vi "Dialog GraphSetting (XY).vi"(11 "XYグラフref(in)":refnum<vi>) -> ()   [LabVIEW 2016]
uses:
  TypeDef/GraphSetting Appearance.ctl
  TypeDef/GraphSetting Plot.ctl
  SupportVIs/GraphSetting Scale.ctl
  TypeDef/GraphSetting DisplayFormatType.ctl
  TypeDef/GraphSetting All.ctl
  TypeDef/GraphSetting Command.ctl
  Library/Event/Write User Event (Array).vi
  <vilib>/Utility/xml.llb/Write to XML File(string).vi
  <vilib>/Utility/xml.llb/Read From XML File(string).vi
  <vilib>/measure/NI_MABase.lvlib
  TypeDef/XYData.ctl
panel:
  out "XYグラフ":cluster{"X":dbl[], "Y":dbl[]}[](graph)
  in  "ファイル読込":bool
  in  "ファイル保存":bool
  in  "タブ制御器":enum32{"外観", "スケール", "プロット"}(tab)
  in  "外観":T1
  in  "Yスケール選択":u16(ring) items=["振幅"]
  in  "スケール(Y軸)":T2
  in  "スケール(X軸)":T2
  in  "Xスケール選択":u16(ring) items=["時間"]
  in  "プロット":T4 {"Yスケール" items=["振幅"]; "Xスケール" items=["時間"]; "プロット補間" max=5 step=1; "ポイントスタイル" max=16 step=1; "太さ" max=5 step=1; "ラインスタイル" max=4 step=1}
  in  "プロット選択":u16(ring) items=["正弦波", "プロット1"]
  in  "停止ボタン":bool
  # "スケールのスタイルとカラー"
  # "スケール係数"
  # "スケールのスタイルとカラー"
  # "スケールのスタイルとカラー"
  # "スケール係数"
  # "スケールのスタイルとカラー"
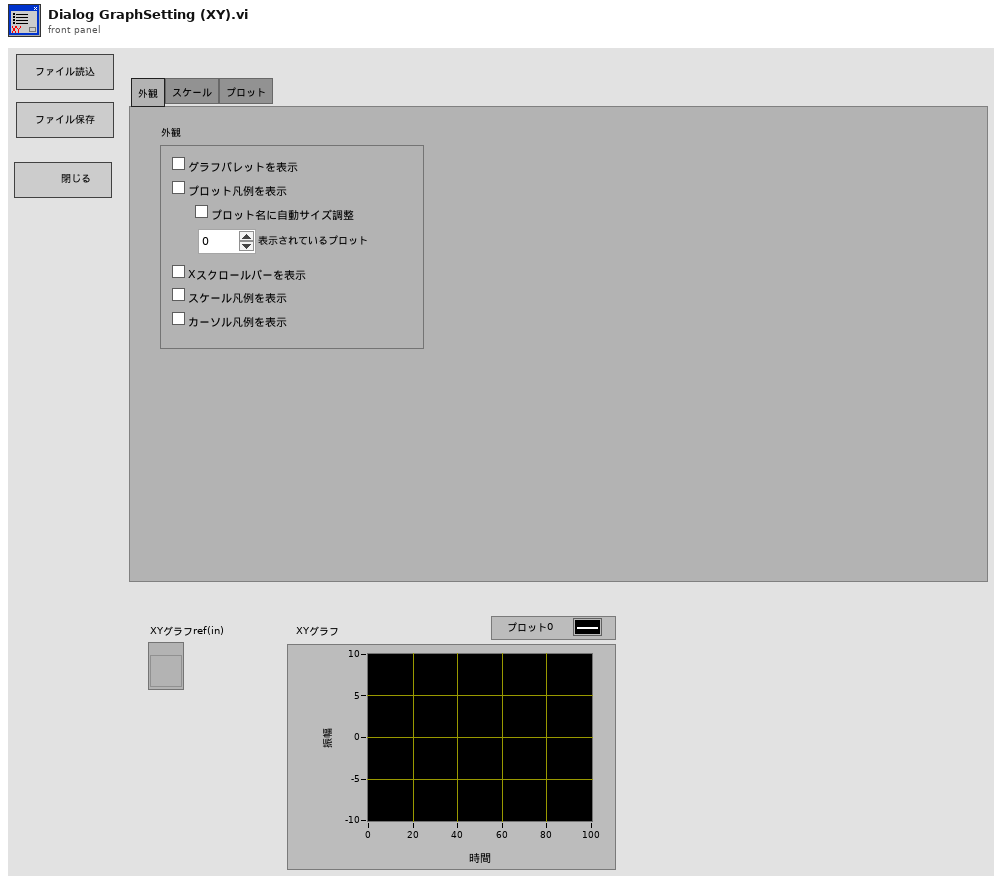
[diagram p1: front panel]
types:
  T1 = typedef "GraphSetting Appearance.ctl" = cluster{"グラフパレットを表示":bool, "プロット凡例を表示":bool, "プロット名に自動サイズ調整":bool, "表示されているプロット":u32, "Xスクロールバーを表示":bool, "スケール凡例を表示":bool, "カーソル凡例を表示":bool}
  T2 = typedef "GraphSetting Scale.ctl" = cluster{"名前":string, "スケールラベルを表示":bool, "スケールを表示":bool, "ログ":bool, "反転":bool, "自動スケール":bool, "最小":dbl, "最大":dbl, "オフセット":dbl, "乗数":dbl, "主目盛り":u32, "補助目盛り":u32, "マーカテキスト":u32, "主グリッド":u32, "補助グリッド":u32, "タイプ":T3, "小数点以下桁数":u8}
  T3 = typedef "GraphSetting DisplayFormatType.ctl" = enum8{"浮動小数点", "科学", "工学", "バイナリ", "８進数", "１６進数", "相対時間", "時間と日時", "SI"}
  T4 = typedef "GraphSetting Plot.ctl" = cluster{"名前":string, "表示":bool, "ラインスタイル":u8, "太さ":u8, "ポイントスタイル":u8, "プロット補間":u8, "ラインカラー":u32, "ポイント/塗りつぶし":u32, "Xスケール":u16, "Yスケール":u16}
  T5 = typedef "XYData.ctl" = cluster{"X":dbl[], "Y":dbl[]}
  T6 = typedef "GraphSetting All.ctl" = cluster{"外観":T1, "スケールX[]":T2[], "スケールY[]":T2[], "プロット[]":T4[]}
  T7 = typedef "GraphSetting Command.ctl" = enum16{"Get(ref->ctl)", "Set(ctl->ref)"}
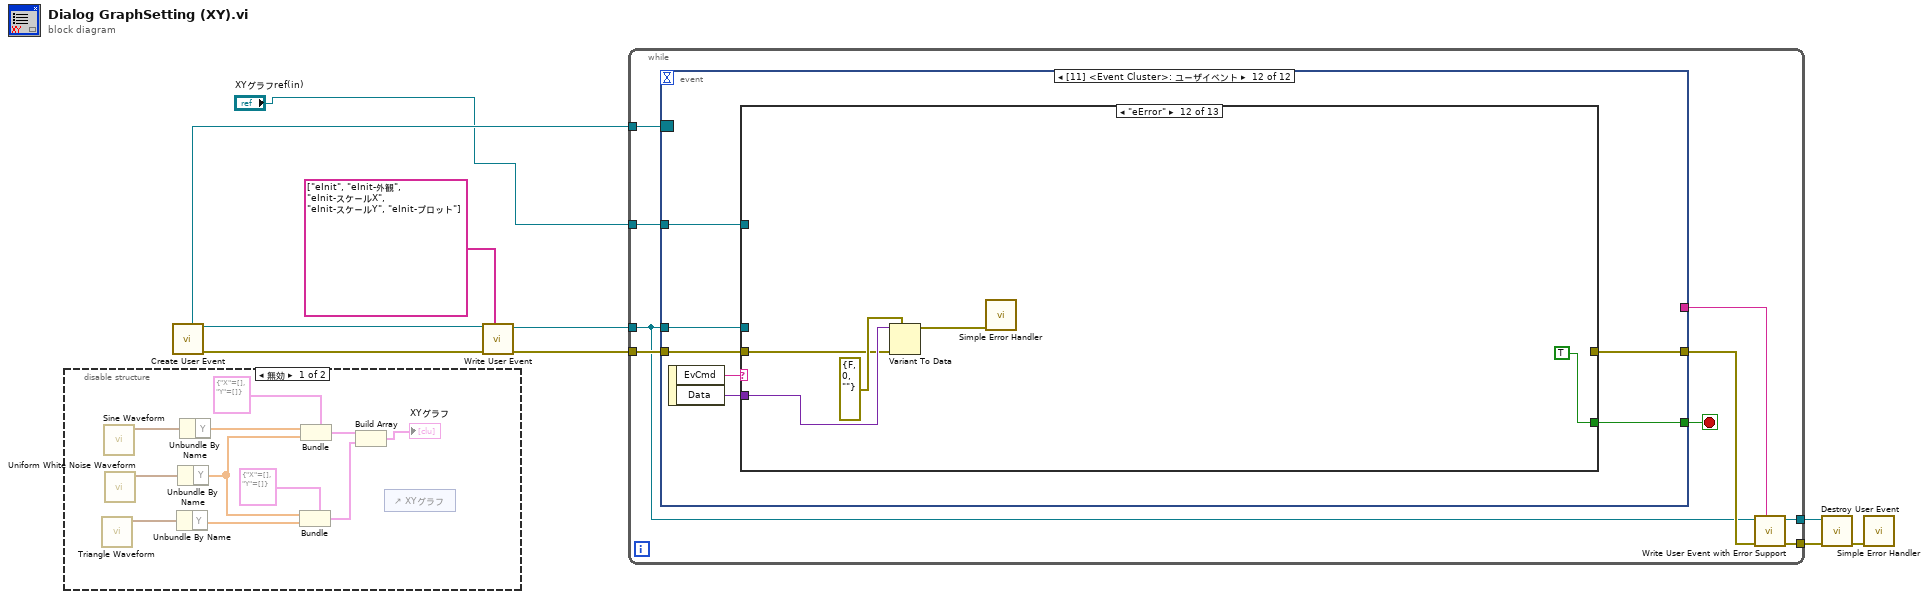
[diagram p0: block diagram]
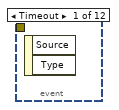
[diagram p3: hidden frame]
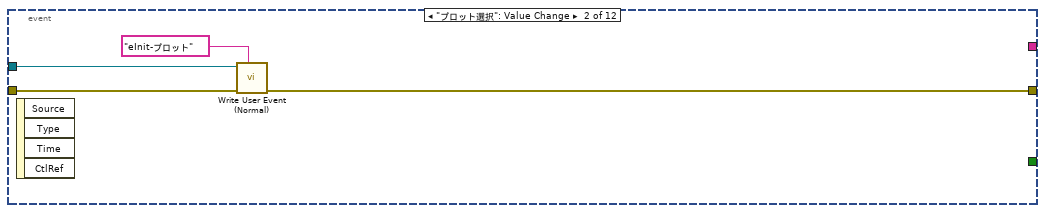
[diagram p4: hidden frame]
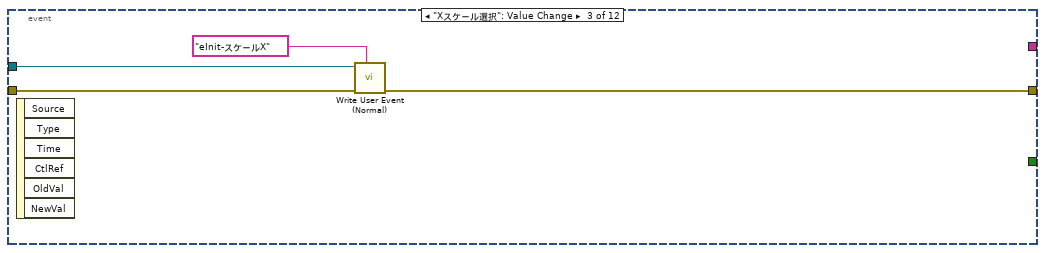
[diagram p5: hidden frame]
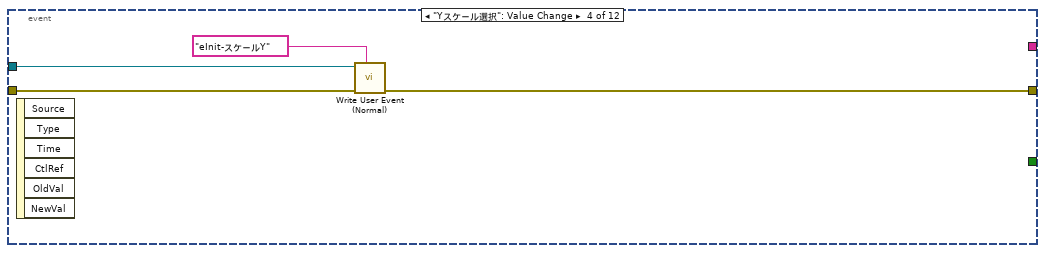
[diagram p6: hidden frame]
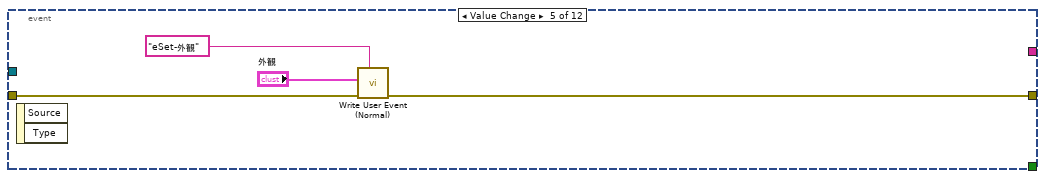
[diagram p7: hidden frame]
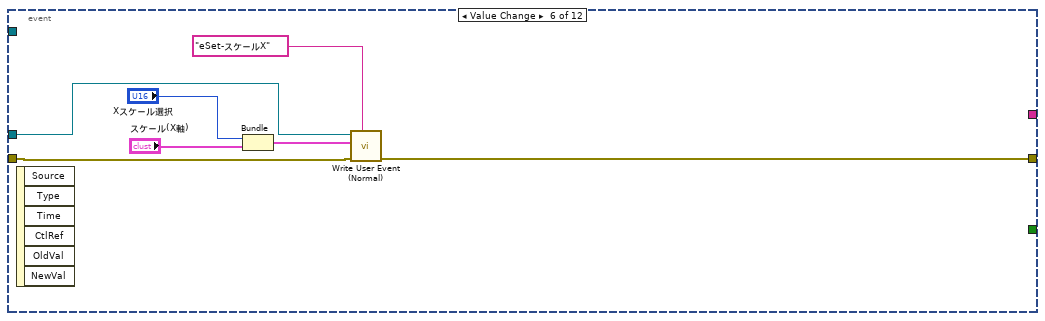
[diagram p8: hidden frame]
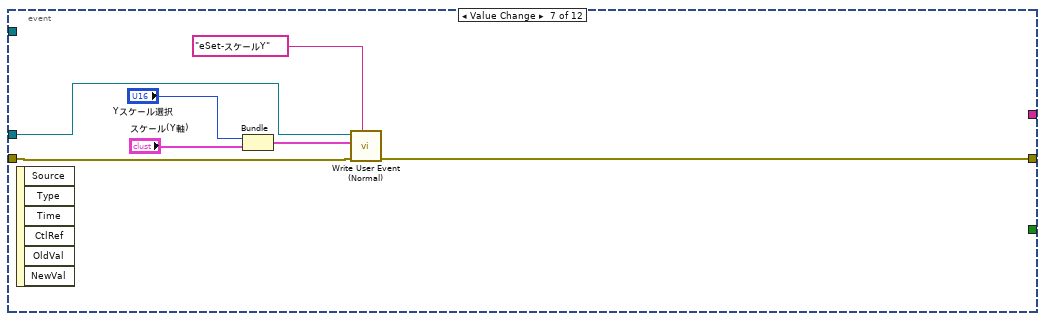
[diagram p9: hidden frame]
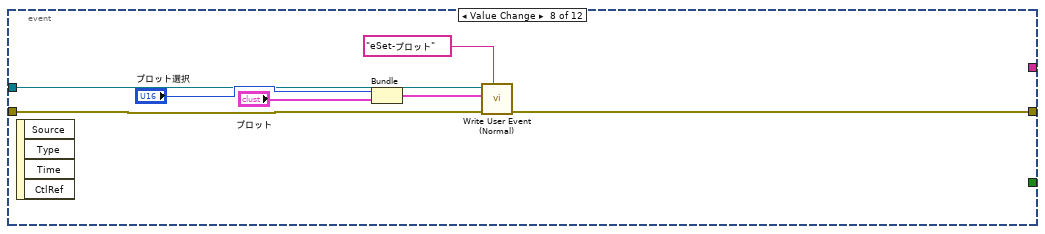
[diagram p10: hidden frame]
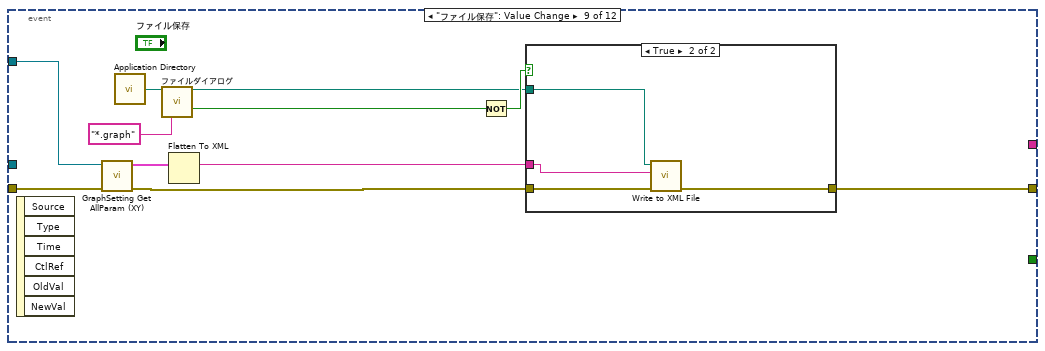
[diagram p11: hidden frame]
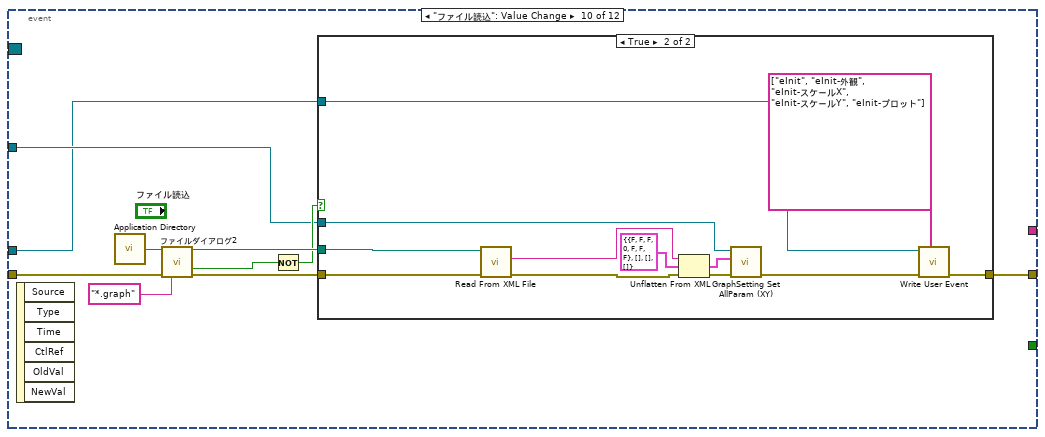
[diagram p13: hidden frame]
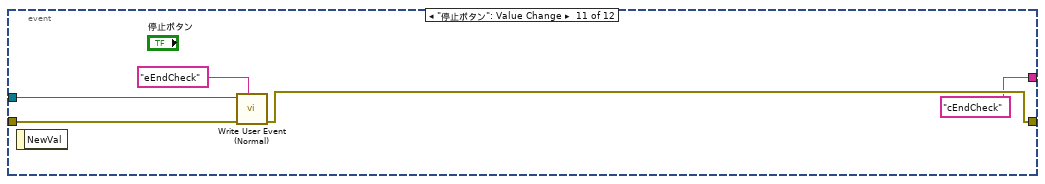
[diagram p15: hidden frame]
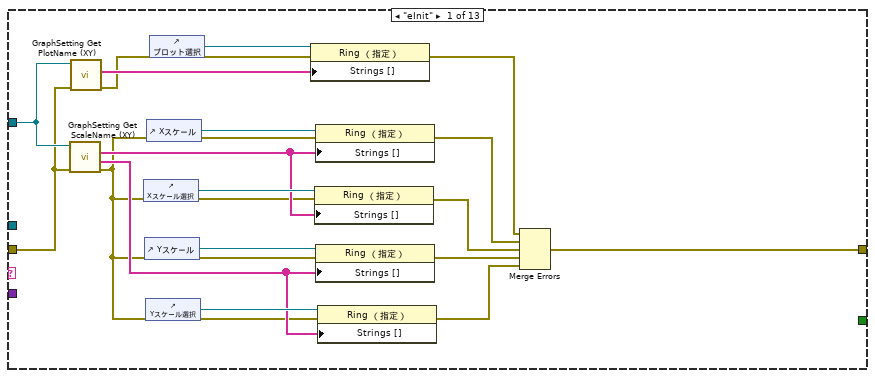
[diagram p16: hidden frame]
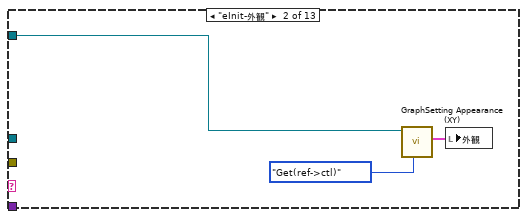
[diagram p17: hidden frame]
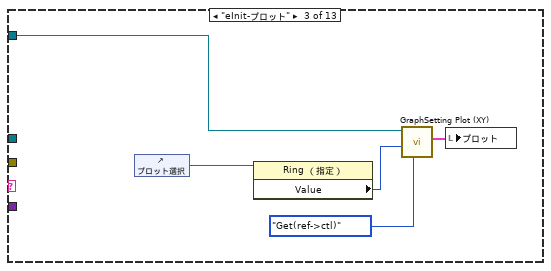
[diagram p18: hidden frame]
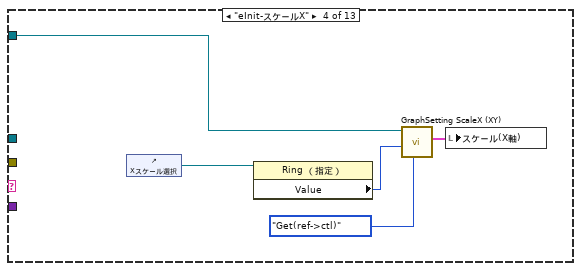
[diagram p19: hidden frame]
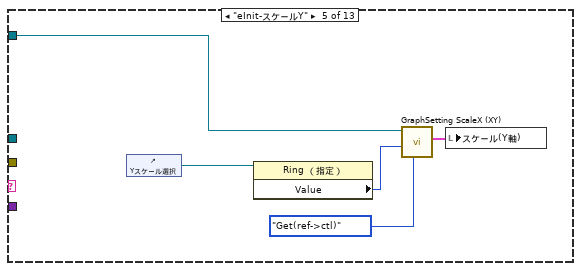
[diagram p20: hidden frame]
diagram:
  n1 = disable-structure shown="無効" {
    frame Disabled {
      n2 = call <vilib>:"Triangle Waveform.vi"() -> ("signal out"=w16:waveform(dbl))  [unwired: 10 in, 1 out]
      n3 = call <vilib>:"Sine Waveform.vi"() -> ("signal out"=w21:waveform(dbl))  [unwired: 10 in, 1 out]
      n4 = call <vilib>:"Uniform White Noise Waveform.vi"() -> ("signal out"=w17:waveform(dbl))  [unwired: 10 in, 1 out]
      n5 = Unbundle By Name(w16) -> ("Y"=w14:dbl[])
      n6 = Unbundle By Name(w17) -> ("Y"=w13:dbl[])
      n7 = Unbundle By Name(w21) -> ("Y"=w18:dbl[])
      n8 = Bundle(cluster=T5 {"X"=[], "Y"=[]} ("XYグラグデータ"), "X"=w13, "Y"=w14) -> (w11:T5)
      n9 = Bundle(cluster=T5 {"X"=[], "Y"=[]} ("XYグラグデータ"), "X"=w18, "Y"=w13) -> (w12:T5)
      n10 = Build Array(w12, w11) -> (→"XYグラフ":T5[])
      n11 = control-ref of="XYグラフ"() -> ()  [unwired: 1 out]
    }
    frame Enabled {
    }
  }
  n12 = call "Create User Event.vi"() -> ("error out"=w8:errorcluster, "User Event"=w9:refnum<user-event>, "Event Registration Refnum"=w10:refnum<event-registration>)  [unwired: 9 in]
  n13 = call-poly "Write User Event.vi"("EvCmd[]"=string[] ["eInit", "eInit-外観", "eInit-スケールX", "eInit-スケールY", "eInit-プロット"], "エラー入力（エラーなし）"=w8, "ユーザイベント入力"=w9) -> ("エラー出力"=w4:errorcluster, "ユーザイベント出力"=w5:refnum<user-event>)  [unwired: 7 in]
  n14 = while {
    tunnel: w4 -> [w29]
    tunnel: w10 -> [w30]
    tunnel: [w26] -> w7
    tunnel: w5 -> [w22]
    tunnel: "XYグラフref(in)" -> [w28]
    tunnel: [w23] -> w2
    stop <- w24 stop-if-true
    n15 = event shown="[11] <Event Cluster>: ユーザイベント" {
      selector: w30 -> [_ _ _ _ _ _ _ _ _ _ _ _]
      dyn-events: _ -> [_ _ _ _ _ _ _ _ _ _ _ _]
      timeout: _ -> [_ _ _ _ _ _ _ _ _ _ _ _]
      tunnel: [_ _ _ _ _ _ _ _ _ _ _ w114] -> w24
      tunnel: [_ w32 w36 w39 w43 w48 w55 w62 w72 w85 w108 w115] -> w27
      tunnel: w29 -> [_ w33 w38 w41 w44 w47 w56 w63 w69 w91 w110 w116]
      tunnel: w22 -> [_ w34 w37 w40 _ w51 w57 w64 _ w84 w111 w113]
      tunnel: w28 -> [_ _ _ _ _ _ _ _ w68 w86 _ w112]
      tunnel: [_ _ _ _ _ _ _ _ _ _ "cEndCheck" _] -> w25
      event Timeout {
        n16 = event-data() -> ()  [unwired: 1 in, 2 out]
      }
      event "プロット選択": Value Change {
        n17 = event-data() -> ()  [unwired: 1 in, 4 out]
        n18 = call "Write User Event (Normal).vi"("EvCmd"="eInit-プロット", "エラー入力（エラーなし）"=w33, "ユーザイベント入力"=w34) -> ("エラー出力"=w32:errorcluster)  [unwired: 7 in, 1 out]
      }
      event "Xスケール選択": Value Change {
        n19 = event-data() -> ()  [unwired: 1 in, 6 out]
        n20 = call "Write User Event (Normal).vi"("EvCmd"="eInit-スケールX", "エラー入力（エラーなし）"=w38, "ユーザイベント入力"=w37) -> ("エラー出力"=w36:errorcluster)  [unwired: 7 in, 1 out]
      }
      event "Yスケール選択": Value Change {
        n21 = event-data() -> ()  [unwired: 1 in, 6 out]
        n22 = call "Write User Event (Normal).vi"("EvCmd"="eInit-スケールY", "エラー入力（エラーなし）"=w41, "ユーザイベント入力"=w40) -> ("エラー出力"=w39:errorcluster)  [unwired: 7 in, 1 out]
      }
      event Value Change {
        n23 = event-data() -> ()  [unwired: 1 in, 2 out]
        n24 = call "Write User Event (Normal).vi"("EvCmd"="eSet-外観", "エラー入力（エラーなし）"=w44, "データ"="外観") -> ("エラー出力"=w43:errorcluster)  [unwired: 7 in, 1 out]
      }
      event Value Change {
        n25 = event-data() -> ()  [unwired: 1 in, 6 out]
        n26 = Bundle("Xスケール選択"="Xスケール選択", "スケール(X軸)"="スケール(X軸)") -> (w52:cluster{"Xスケール選択":u16, "スケール(X軸)":T2})  [unwired: 1 in]
        n27 = call "Write User Event (Normal).vi"("EvCmd"="eSet-スケールX", "エラー入力（エラーなし）"=w47, "データ"=w52, "ユーザイベント入力"=w51) -> ("エラー出力"=w48:errorcluster)  [unwired: 6 in, 1 out]
      }
      event Value Change {
        n28 = event-data() -> ()  [unwired: 1 in, 6 out]
        n29 = Bundle("Yスケール選択"="Yスケール選択", "スケール(Y軸)"="スケール(Y軸)") -> (w58:cluster{"Yスケール選択":u16, "スケール(Y軸)":T2})  [unwired: 1 in]
        n30 = call "Write User Event (Normal).vi"("EvCmd"="eSet-スケールY", "エラー入力（エラーなし）"=w56, "データ"=w58, "ユーザイベント入力"=w57) -> ("エラー出力"=w55:errorcluster)  [unwired: 6 in, 1 out]
      }
      event Value Change {
        n31 = event-data() -> ()  [unwired: 1 in, 4 out]
        n32 = Bundle("プロット選択"="プロット選択", "プロット"="プロット") -> (w65:cluster{"プロット選択":u16, "プロット":T4})  [unwired: 1 in]
        n33 = call "Write User Event (Normal).vi"("EvCmd"="eSet-プロット", "エラー入力（エラーなし）"=w63, "データ"=w65, "ユーザイベント入力"=w64) -> ("エラー出力"=w62:errorcluster)  [unwired: 6 in, 1 out]
      }
      event "ファイル保存": Value Change {
        n34 = event-data() -> ()  [unwired: 1 in, 6 out]
        n35 = call "GraphSetting Get AllParam (XY).vi"("エラー入力（エラーなし）"=w69, "XYグラフref(in)"=w68) -> ("エラー出力"=w71:errorcluster, "クラスタ"=w70:cluster{"外観(out)":T1, T2[], T2[], T4[]})  [unwired: 8 in]
        n36 = call <vilib>:"Application Directory.vi"() -> ("Application Directory"=w77:path)
        n37 = call "ファイルダイアログ"("start path"=w77, "pattern (all files)"="*.graph") -> ("selected path"=w73:path, "cancelled"=w74:bool)  [unwired: 10 in, 2 out]
        n38 = Flatten To XML(anything=w70) -> (xml string=w75:string)
        n39 = Not(x=w74) -> (.not. x?=w76:bool)
        n40 = case shown="TRUE" w76 {
          tunnel: w73 -> [_ w83]
          tunnel: w75 -> [_ w82]
          tunnel: w71 -> [w79 w80]
          tunnel: [w79 w81] -> w72
          frame False {
          }
          frame True {
            n41 = call-poly <vilib>:"Write to XML File.vi"("error in (no error)"=w80, "XML Input"=w82, "XML File Path"=w83) -> ("error out"=w81:errorcluster)  [unwired: 6 in, 2 out]
          }
        }
      }
      event "ファイル読込": Value Change {
        n42 = event-data() -> ()  [unwired: 1 in, 6 out]
        n43 = call <vilib>:"Application Directory.vi"() -> ("Application Directory"=w93:path)
        n44 = call "ファイルダイアログ2"("start path"=w93, "error in"=w91, "pattern (all files)"="*.graph") -> ("selected path"=w90:path, "cancelled"=w89:bool, "error out"=w87:errorcluster)  [unwired: 9 in, 1 out]
        n45 = Not(x=w89) -> (.not. x?=w88:bool)
        n46 = case shown="TRUE" w88 {
          tunnel: w90 -> [_ w104]
          tunnel: w87 -> [w94 w102]
          tunnel: w86 -> [_ w99]
          tunnel: [w94 w96] -> w85
          tunnel: w84 -> [_ w98]
          frame False {
          }
          frame True {
            n47 = call-poly <vilib>:"Read From XML File.vi"("error in (no error)"=w102, "XML File Path"=w104) -> ("error out"=w103:errorcluster, "XML Elements"=w105:string)  [unwired: 7 in, 1 out]
            n48 = Unflatten From XML(xml string=w105, type=T6 {"外観"={"グラフパレットを表示"=FALSE, "プロット凡例を表示"=FALSE, "プロット名に自動サイズ調整"=FALSE, "表示されているプロット"=0, "Xスクロールバーを表示"=FALSE, "スケール凡例を表示"=FALSE, "カーソル凡例を表示"=FALSE}, "スケールX[]"=[], "スケールY[]"=[], "プロット[]"=[]} ("出力クラスタ"), error in (no error)=w103) -> (value=w101:T6, error out=w100:errorcluster)
            n49 = call "GraphSetting Set AllParam (XY).vi"("error in (no error)"=w100, "Chartグラフパラメータ"=w101, "XYグラフref(in)"=w99) -> ("error out"=w97:errorcluster)  [unwired: 8 in]
            n50 = call-poly "Write User Event.vi"("EvCmd[]"=string[] ["eInit", "eInit-外観", "eInit-スケールX", "eInit-スケールY", "eInit-プロット"], "エラー入力（エラーなし）"=w97, "ユーザイベント入力"=w98) -> ("エラー出力"=w96:errorcluster)  [unwired: 7 in, 1 out]
          }
        }
      }
      event "停止ボタン": Value Change {
        n51 = event-data() -> ()  [unwired: 1 in, 1 out]
        n52 = call "Write User Event (Normal).vi"("EvCmd"="eEndCheck", "エラー入力（エラーなし）"=w110, "ユーザイベント入力"=w111) -> ("エラー出力"=w108:errorcluster)  [unwired: 7 in, 1 out]
      }
      event User Event {
        n53 = event-data() -> ("EvCmd"=w118:string, "Data"=w117:variant)  [unwired: 1 in]
        n54 = case shown="\"eError\"" w118 {
          selector: w118 -> [_ _ _ _ _ _ _ _ _ _ _ _ w202]
          tunnel: w117 -> [_ _ _ _ _ w159 w167 w178 w188 _ _ w201 _]
          tunnel: w116 -> [w128 _ _ _ _ w157 w169 w177 w187 w192 w196 w199 _]
          tunnel: [w119 _ _ _ _ w155 w162 w171 w181 w191 w196 _ _] -> w115
          tunnel: [_ _ _ _ _ _ _ _ _ _ TRUE TRUE _] -> w114
          tunnel: w113 -> [_ _ _ _ _ _ _ _ _ w194 _ _ _]
          tunnel: w112 -> [w131 w139 w144 w149 w154 w160 w163 w175 w185 _ _ _ _]
          frame "eInit" {
            n55 = call "GraphSetting Get ScaleName (XY).vi"("error in (no error)"=w128, "XYグラフref(in)"=w131) -> ("error out"=w125:errorcluster, "Y軸名称[]"=w127:string[], "X軸名称[]"=w134:string[])  [unwired: 7 in]
            n56 = call "GraphSetting Get PlotName (XY).vi"("error in (no error)"=w128, "XYグラフref(in)"=w131) -> ("error out"=w126:errorcluster, "プロット名称[]"=w129:string[])  [unwired: 8 in]
            n57 = control-ref of="Xスケール選択"() -> (w135:refnum<vi>)
            n58 = control-ref of="Yスケール"() -> (w132:refnum<vi>)
            n59 = control-ref of="Yスケール選択"() -> (w133:refnum<vi>)
            n60 = control-ref of="Xスケール"() -> (w136:refnum<vi>)
            n61 = control-ref of="プロット選択"() -> (w130:refnum<vi>)
            n62 = property class="Ring （指定）"(reference=w130, error in=w126, "Strings []"=w129) -> (error out=w124:errorcluster)  [unwired: 1 out]
            n63 = property class="Ring （指定）"(reference=w135, error in=w125, "Strings []"=w134) -> (error out=w122:errorcluster)  [unwired: 1 out]
            n64 = property class="Ring （指定）"(reference=w136, error in=w125, "Strings []"=w134) -> (error out=w123:errorcluster)  [unwired: 1 out]
            n65 = property class="Ring （指定）"(reference=w132, error in=w125, "Strings []"=w127) -> (error out=w121:errorcluster)  [unwired: 1 out]
            n66 = property class="Ring （指定）"(reference=w133, error in=w125, "Strings []"=w127) -> (error out=w120:errorcluster)  [unwired: 1 out]
            n67 = Merge Errors(w124, w123, w122, w121, w120) -> (w119:errorcluster)
          }
          frame "eInit-外観" {
            n68 = call "GraphSetting Appearance (XY).vi"("コマンド"=GraphSetting_Command."Get(ref->ctl)", "XYグラフref(in)"=w139) -> ("外観(out)"=w138:T1)  [unwired: 8 in, 1 out]
            n69 = local write "外観"(w138) -> ()
          }
          frame "eInit-プロット" {
            n70 = control-ref of="プロット選択"() -> (w143:refnum<vi>)
            n71 = property class="Ring （指定）"(reference=w143) -> ("Value"=w142:u16)  [unwired: 1 in, 2 out]
            n72 = call "GraphSetting Plot (XY).vi"("コマンド"=GraphSetting_Command."Get(ref->ctl)", "アクティブプロット"=w142, "XYグラフref(in)"=w144) -> ("プロット(out)"=w140:T4)  [unwired: 7 in, 1 out]
            n73 = local write "プロット"(w140) -> ()
          }
          frame "eInit-スケールX" {
            n74 = control-ref of="Xスケール選択"() -> (w148:refnum<vi>)
            n75 = property class="Ring （指定）"(reference=w148) -> ("Value"=w147:u16)  [unwired: 1 in, 2 out]
            n76 = call "GraphSetting ScaleX (XY).vi"("コマンド"=GraphSetting_Command."Get(ref->ctl)", "アクティブスケール(X)"=w147, "XYグラフref(in)"=w149) -> ("スケール(out)"=w145:T2)  [unwired: 7 in, 1 out]
            n77 = local write "スケール(X軸)"(w145) -> ()
          }
          frame "eInit-スケールY" {
            n78 = control-ref of="Yスケール選択"() -> (w153:refnum<vi>)
            n79 = property class="Ring （指定）"(reference=w153) -> ("Value"=w152:u16)  [unwired: 1 in, 2 out]
            n80 = call "GraphSetting ScaleX (XY).vi"("コマンド"=GraphSetting_Command."Get(ref->ctl)", "アクティブスケール(X)"=w152, "XYグラフref(in)"=w154) -> ("スケール(out)"=w150:T2)  [unwired: 7 in, 1 out]
            n81 = local write "スケール(Y軸)"(w150) -> ()
          }
          frame "eSet-外観" {
            n82 = Variant To Data(error in=w157, Variant=w159) -> (data=w158:T1, error out=w156:errorcluster)  [unwired: 1 in]
            n83 = call "GraphSetting Appearance (XY).vi"("コマンド"=GraphSetting_Command."Set(ctl->ref)", "error in (no error)"=w156, "外観(in)"=w158, "XYグラフref(in)"=w160) -> ("error out"=w155:errorcluster)  [unwired: 6 in, 1 out]
          }
          frame "eSet-スケールX" {
            n84 = Variant To Data(type=cluster{"Xスケール選択":u16, "スケール(X軸)":T2} {"Xスケール選択"=0, "スケール(X軸)"={"名前"="", "スケールラベルを表示"=FALSE, "スケールを表示"=FALSE, "ログ"=FALSE, "反転"=FALSE, "自動スケール"=FALSE, "最小"=0.0, "最大"=0.0, "オフセット"=0.0, "乗数"=0.0, "主目盛り"=0, "補助目盛り"=0, "マーカテキスト"=0, "主グリッド"=0, "補助グリッド"=0, "タイプ"=enum."浮動小数点", "小数点以下桁数"=0}} ("出力クラスタ"), Variant=w167) -> (data=w166:cluster{"Xスケール選択":u16, "スケール(X軸)":T2})  [unwired: 1 in, 1 out]
            n85 = Unbundle(w166) -> ("Xスケール選択"=w164:u16, "スケール(X軸)"=w165:T2)
            n86 = call "GraphSetting ScaleX (XY).vi"("コマンド"=GraphSetting_Command."Set(ctl->ref)", "error in (no error)"=w169, "アクティブスケール(X)"=w164, "スケール(in)"=w165, "XYグラフref(in)"=w163) -> ("error out"=w162:errorcluster)  [unwired: 5 in, 1 out]
          }
          frame "eSet-スケールY" {
            n87 = Variant To Data(error in=w177, type=cluster{"Xスケール選択":u16, "スケール(X軸)":T2} {"Xスケール選択"=0, "スケール(X軸)"={"名前"="", "スケールラベルを表示"=FALSE, "スケールを表示"=FALSE, "ログ"=FALSE, "反転"=FALSE, "自動スケール"=FALSE, "最小"=0.0, "最大"=0.0, "オフセット"=0.0, "乗数"=0.0, "主目盛り"=0, "補助目盛り"=0, "マーカテキスト"=0, "主グリッド"=0, "補助グリッド"=0, "タイプ"=enum."浮動小数点", "小数点以下桁数"=0}} ("出力クラスタ"), Variant=w178) -> (data=w176:cluster{"Xスケール選択":u16, "スケール(X軸)":T2}, error out=w172:errorcluster)
            n88 = Unbundle(w176) -> ("Xスケール選択"=w173:u16, "スケール(X軸)"=w174:T2)
            n89 = call "GraphSetting ScaleY (XY).vi"("コマンド"=GraphSetting_Command."Set(ctl->ref)", "error in (no error)"=w172, "アクティブスケールY"=w173, "スケール(in)"=w174, "XYグラフref(in)"=w175) -> ("error out"=w171:errorcluster)  [unwired: 5 in, 1 out]
          }
          frame "eSet-プロット" {
            n90 = control-ref of="XYグラフ"() -> ()  [unwired: 1 out]
            n91 = Variant To Data(error in=w187, type=cluster{"プロット選択":u16, "プロット":T4} {"プロット選択"=0, "プロット"={"名前"="", "表示"=FALSE, "ラインスタイル"=0, "太さ"=0, "ポイントスタイル"=0, "プロット補間"=0, "ラインカラー"=0, "ポイント/塗りつぶし"=0, "Xスケール"=0, "Yスケール"=0}} ("出力クラスタ"), Variant=w188) -> (data=w186:cluster{"プロット選択":u16, "プロット":T4}, error out=w184:errorcluster)
            n92 = Unbundle(w186) -> ("プロット選択"=w183:u16, "プロット"=w182:T4)
            n93 = call "GraphSetting Plot (XY).vi"("コマンド"=GraphSetting_Command."Set(ctl->ref)", "error in (no error)"=w184, "アクティブプロット"=w183, "プロット(in)"=w182, "XYグラフref(in)"=w185) -> ("error out"=w181:errorcluster)  [unwired: 5 in, 1 out]
          }
          frame "eEndCheck" {
            n94 = call "Write User Event (Normal).vi"("EvCmd"="eEnd", "エラー入力（エラーなし）"=w192, "ユーザイベント入力"=w194) -> ("エラー出力"=w191:errorcluster)  [unwired: 7 in, 1 out]
          }
          frame "eEnd" {
          }
          frame "eError" {
            n95 = Variant To Data(error in=w199, type=errorcluster {"status"=FALSE, "code"=0, "source"=""} ("エラー定数"), Variant=w201) -> (data=w198:errorcluster)  [unwired: 1 out]
            n96 = call <vilib>:"Simple Error Handler.vi"("error in (no error)"=w198) -> ()  [unwired: 4 in, 5 out]
          }
          frame Default {
            n97 = call "DialogProgramError.vi"("エラー内容"="ユーザイベント例外" ("エラー詳細"), "エラー詳細"=w202) -> ()  [unwired: 9 in, 1 out]
          }
        }
      }
    }
    n98 = call "Write User Event with Error Support.vi"("EvCmd"=w25, "エラー入力（エラーなし）"=w27, "ユーザイベント入力"=w22) -> ("エラー出力"=w26:errorcluster, "ユーザイベント出力"=w23:refnum<user-event>)  [unwired: 7 in]
  }
  n99 = call "Destroy User Event.vi"("error in (no error)"=w7, "User Event"=w2) -> ("error out"=w6:errorcluster)  [unwired: 9 in]
  n100 = call <vilib>:"Simple Error Handler.vi"("error in (no error)"=w6) -> ()  [unwired: 4 in, 5 out]
